vi "DAQmx_SyncAll.vi"(8 "error in (no error)":errorcluster, 11 "Array in":refnum<class "DAQmx.lvclass">[](array[class])) -> (0 "error out":errorcluster, 3 "Array out":refnum<class "DAQmx.lvclass">[](array[class]))   [LabVIEW 2016, in "DAQmx.lvclass"]
uses:
  DAQmx.lvclass
  DAQmx.lvclass/DAQmx.ctl
  <vilib>/DAQmx/configure/trigger.llb/DAQmx Start Trigger (Digital Edge).vi
  <resource>/objmgr/daqmx.rc
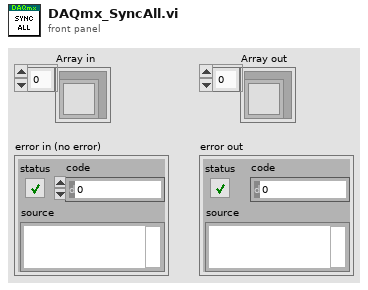
[diagram p1: front panel]
types:
  T1 = cluster{"RefClk.Src":tag, "SyncPulse.src":tag, "StartTrigger.src":tag, "SyncPulse.SyncTime":dbl}
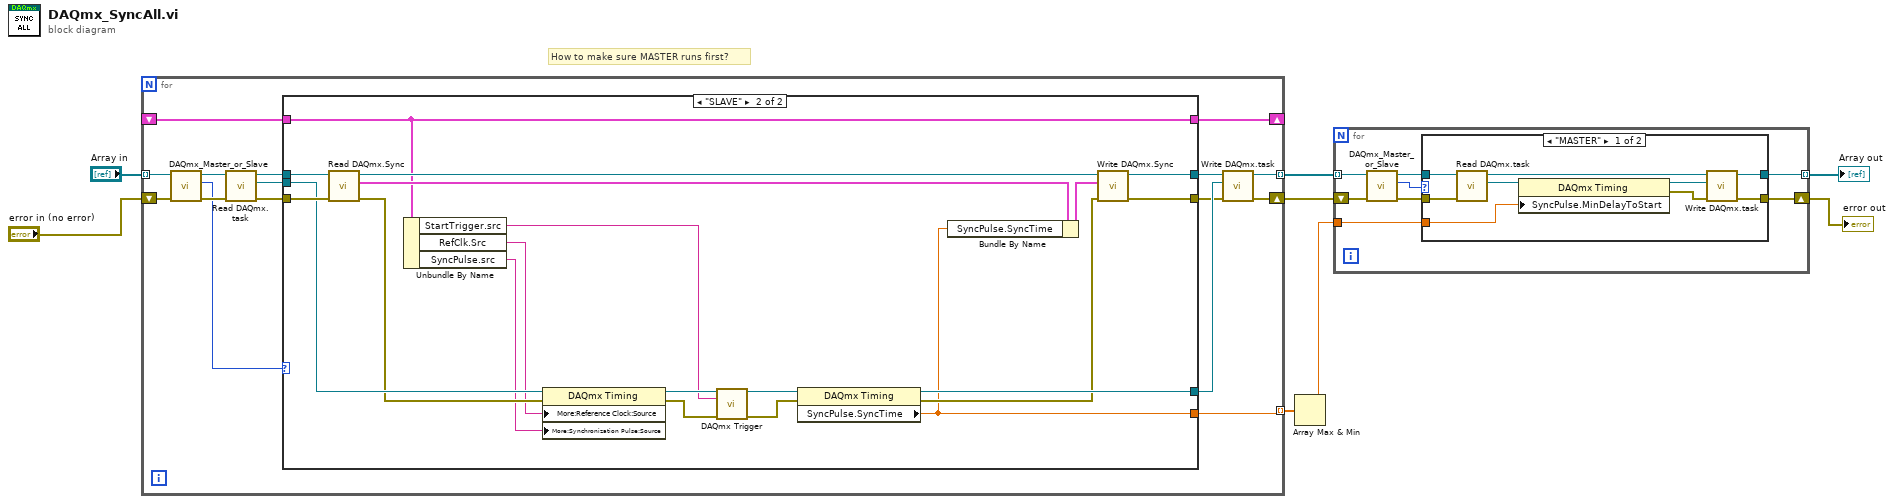
[diagram p0: block diagram]
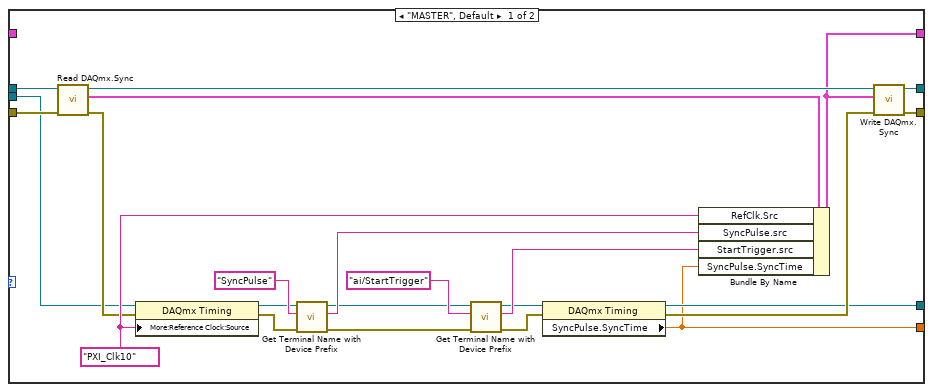
[diagram p2: hidden frame]
diagram:
  # "How to make sure MASTER runs first?"
  n1 = for {
    tunnel: "Array in" -> [w15] mode=indexing
    shift-right: [w13] -> w4
    shift-left: "error in (no error)" -> [w14]
    tunnel: [w12] -> w5 mode=indexing
    tunnel: [w11] -> w3 mode=indexing
    shift-right: [w10] -> _
    shift-left: _ -> [w9]
    n2 = call "DAQmx_Master_or_Slave.vi"("error in (no error)"=w14, "DAQmx in"=w15) -> ("error out"=w18:errorcluster, "Enum"=w16:enum16{"MASTER", "SLAVE"}, "DAQmx out"=w17:refnum<class "DAQmx.lvclass">)  [unwired: 7 in]
    n3 = call "Read DAQmx.task.vi"("error in (no error)"=w18, "DAQmx in"=w17) -> ("error out"=w20:errorcluster, "task"=w24:refnum<k21>, "DAQmx out"=w22:refnum<class "DAQmx.lvclass">)  [unwired: 7 in]
    n4 = case shown="\"SLAVE\"" w16 {
      tunnel: w24 -> [w29 w63]
      tunnel: [w27 w51] -> w23
      tunnel: w20 -> [w33 w64]
      tunnel: w22 -> [w36 w67]
      tunnel: [w34 w66] -> w21
      tunnel: [w30 w53] -> w19
      tunnel: [w26 w49] -> w12
      tunnel: [w25 w48] -> w10
      tunnel: w9 -> [_ w48]
      frame "MASTER", Default {
        w38 = tag "PXI_Clk10" ("RefClk.Src")
        n5 = call "Read DAQmx.Sync.vi"("error in (no error)"=w33, "DAQmx in"=w36) -> ("error out"=w32:errorcluster, "Sync"=w31:T1, "DAQmx out"=w35:refnum<class "DAQmx.lvclass">)  [unwired: 7 in]
        n6 = property class="DAQmx Timing"(reference=w29, error in=w32, "More:Reference Clock:Source"=w38) -> (reference out=w45:refnum<k21>, error out=w44:errorcluster)
        n7 = call "Get Terminal Name with Device Prefix.vi"("error in (no error)"=w44, "Local Terminal Name"="SyncPulse", "task/channels in"=w45) -> ("error out"=w41:errorcluster, "Terminal Name with Device Prefix"=w43:tag, "task out"=w42:refnum<k21>)  [unwired: 6 in]
        n8 = call "Get Terminal Name with Device Prefix.vi"("error in (no error)"=w41, "Local Terminal Name"="ai/StartTrigger", "task/channels in"=w42) -> ("error out"=w37:errorcluster, "Terminal Name with Device Prefix"=w40:tag, "task out"=w39:refnum<k21>)  [unwired: 6 in]
        n9 = property class="DAQmx Timing"(reference=w39, error in=w37) -> (reference out=w27:refnum<k21>, error out=w28:errorcluster, "SyncPulse.SyncTime"=w26:dbl)
        n10 = Bundle By Name(cluster=w31, "RefClk.Src"=w38, "SyncPulse.src"=w43, "StartTrigger.src"=w40, "SyncPulse.SyncTime"=w26) -> (w25:T1)
        n11 = call "Write DAQmx.Sync.vi"("error in (no error)"=w28, "Sync"=w25, "DAQmx in"=w35) -> ("error out"=w30:errorcluster, "DAQmx out"=w34:refnum<class "DAQmx.lvclass">)  [unwired: 7 in]
      }
      frame "SLAVE" {
        n12 = call "Read DAQmx.Sync.vi"("error in (no error)"=w64, "DAQmx in"=w67) -> ("error out"=w62:errorcluster, "Sync"=w54:T1, "DAQmx out"=w65:refnum<class "DAQmx.lvclass">)  [unwired: 7 in]
        n13 = Unbundle By Name(w48) -> ("StartTrigger.src"=w52:tag, "RefClk.Src"=w57:tag, "SyncPulse.src"=w56:tag)
        n14 = property class="DAQmx Timing"(reference=w63, error in=w62, "More:Reference Clock:Source"=w57, "More:Synchronization Pulse:Source"=w56) -> (reference out=w60:refnum<k21>, error out=w61:errorcluster)
        n15 = call-poly <vilib>:"DAQmx Trigger.vi"("task/channels in"=w60, "source"=w52, "error in"=w61) -> ("task out"=w59:refnum<k21>, "error out"=w58:errorcluster)  [unwired: 11 in]
        n16 = property class="DAQmx Timing"(reference=w59, error in=w58) -> (reference out=w51:refnum<k21>, error out=w50:errorcluster, "SyncPulse.SyncTime"=w49:dbl)
        n17 = Bundle By Name(cluster=w54, "SyncPulse.SyncTime"=w49) -> (w55:T1)
        n18 = call "Write DAQmx.Sync.vi"("error in (no error)"=w50, "Sync"=w55, "DAQmx in"=w65) -> ("error out"=w53:errorcluster, "DAQmx out"=w66:refnum<class "DAQmx.lvclass">)  [unwired: 7 in]
      }
    }
    n19 = call "Write DAQmx.task.vi"("error in (no error)"=w19, "task"=w23, "DAQmx in"=w21) -> ("error out"=w13:errorcluster, "DAQmx out"=w11:refnum<class "DAQmx.lvclass">)  [unwired: 7 in]
  }
  n20 = Array Max & Min(array=w5) -> (max value=w2:dbl)  [unwired: 3 out]
  n21 = for {
    tunnel: w2 -> [w70]
    tunnel: w3 -> [w75] mode=indexing
    tunnel: [w69] -> w8 mode=indexing
    shift-right: [w68] -> w7
    shift-left: w4 -> [w74]
    n22 = call "DAQmx_Master_or_Slave.vi"("error in (no error)"=w74, "DAQmx in"=w75) -> ("error out"=w71:errorcluster, "Enum"=w73:enum16{"MASTER", "SLAVE"}, "DAQmx out"=w72:refnum<class "DAQmx.lvclass">)  [unwired: 7 in]
    n23 = case shown="\"MASTER\"" w73 {
      tunnel: w72 -> [w84 w86]
      tunnel: w71 -> [w83 w85]
      tunnel: w70 -> [w79 _]
      tunnel: [w77 w86] -> w69
      tunnel: [w76 w85] -> w68
      frame "MASTER" {
        n24 = call "Read DAQmx.task.vi"("error in (no error)"=w83, "DAQmx in"=w84) -> ("task"=w82:refnum<k21>, "DAQmx out"=w80:refnum<class "DAQmx.lvclass">)  [unwired: 7 in, 1 out]
        n25 = property class="DAQmx Timing"(reference=w82, "SyncPulse.MinDelayToStart"=w79) -> (reference out=w81:refnum<k21>, error out=w78:errorcluster)  [unwired: 1 in]
        n26 = call "Write DAQmx.task.vi"("error in (no error)"=w78, "task"=w81, "DAQmx in"=w80) -> ("error out"=w76:errorcluster, "DAQmx out"=w77:refnum<class "DAQmx.lvclass">)  [unwired: 7 in]
      }
      frame "SLAVE", Default {
      }
    }
  }
  "error out" <- w7
  "Array out" <- w8
